vi "Pressure_Test_V2.vi"() -> ()   [LabVIEW 2015]
uses:
  <vilib>/Waveform/WDTOps.llb/WDT Append Waveforms DBL.vi
  <vilib>/Waveform/WDTOps.llb/WDT Waveform Duration DBL.vi
panel:
  in  "Stop Duration":dbl
  out "Current Duration":dbl format="%0.2f"
  out "Waveform Chart 1":dynamicdata(graph)
  in  "Enable":bool=TRUE
  in  "Filename":path=path "VehicleAccerometer/Front_Left_ACC.lvm"
  in  "Data Collection":bool
  in  "number of samples":i32=800
  in  "rate":dbl=2000.0
  # "256"
  # "512"
  # "Accelerometer Settings"
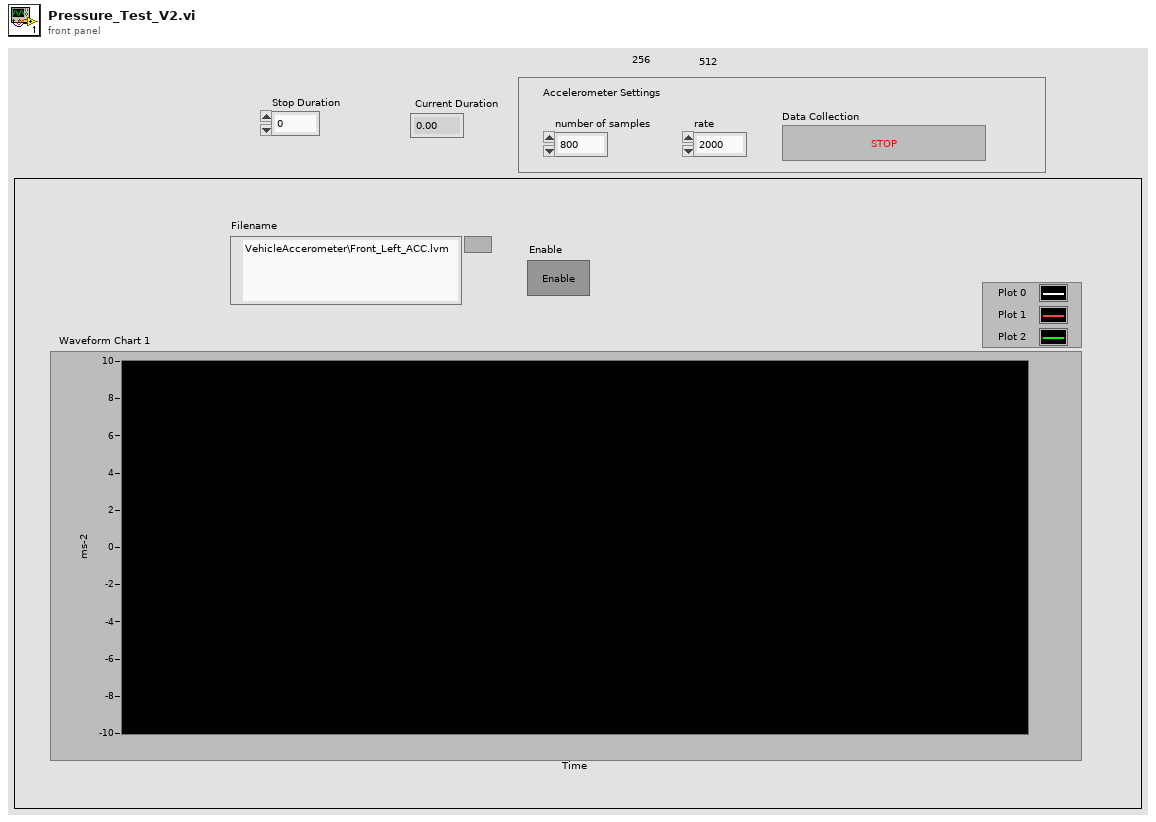
[diagram p1: front panel]
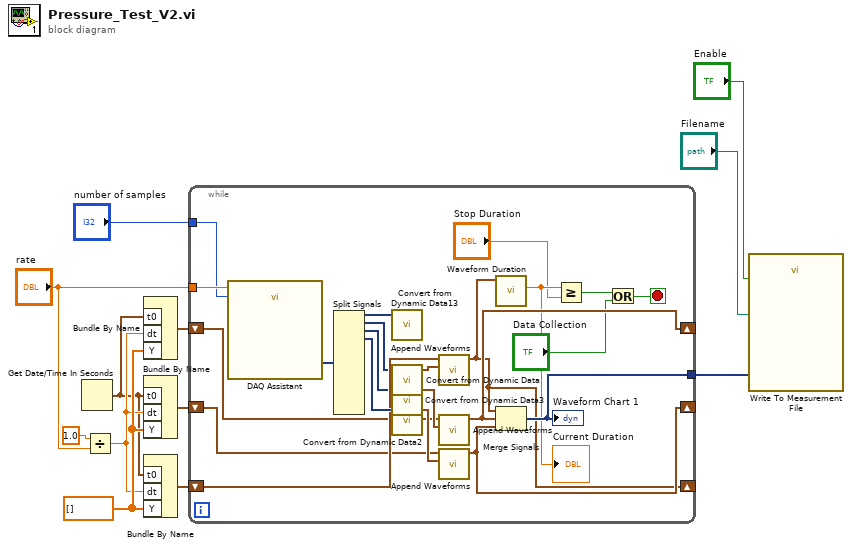
[diagram p0: block diagram]
diagram:
  w3 = dbl[] [] ("Y")
  n1 = Get Date/Time In Seconds() -> (seconds since 1Jan1904=w1:timestamp)
  n2 = Divide(x=1.0, y="rate") -> (x/y=w2:dbl)
  n3 = Bundle By Name("t0"=w1, "dt"=w2, "Y"=w3) -> (w12:waveform(dbl))  [unwired: 1 in]
  n4 = Bundle By Name("t0"=w1, "dt"=w2, "Y"=w3) -> (w9:waveform(dbl))  [unwired: 1 in]
  n5 = Bundle By Name("t0"=w1, "dt"=w2, "Y"=w3) -> (w8:waveform(dbl))  [unwired: 1 in]
  n6 = while {
    shift-right: [w23] -> _
    shift-left: w12 -> [w25]
    tunnel: "rate" -> [w31]
    shift-right: [w22] -> _
    shift-left: w9 -> [w24]
    shift-right: [w15] -> _
    shift-left: w8 -> [w28]
    tunnel: [w21] -> w5
    tunnel: "number of samples" -> [w14]
    stop <- w16 stop-if-true
    n7 = call "DAQ Assistant"("rate"=w31, "number of samples"=w14) -> ("data"=w30:dynamicdata)  [unwired: 15 in, 2 out]
    n8 = Split Signals(w30) -> (w13:dynamicdata, w26:dynamicdata, w27:dynamicdata, w34:dynamicdata)  [unwired: 13 in, 9 out]
    n9 = call "Convert from Dynamic Data13"("Dynamic Data Type"=w13) -> ()  [unwired: 3 in, 1 out]
    n10 = call "Convert from Dynamic Data"("Dynamic Data Type"=w26) -> ("Waveform"=w29:waveform(dbl))  [unwired: 3 in]
    n11 = call "Convert from Dynamic Data3"("Dynamic Data Type"=w27) -> ("Waveform"=w33:waveform(dbl))  [unwired: 3 in]
    n12 = call "Convert from Dynamic Data2"("Dynamic Data Type"=w34) -> ("Waveform"=w32:waveform(dbl))  [unwired: 3 in]
    n13 = call-poly <vilib>:"Append Waveforms.vi"("waveform B"=w29, "waveform A"=w28) -> ("waveform out"=w15:waveform(dbl))  [unwired: 8 in, 1 out]
    n14 = call-poly <vilib>:"Append Waveforms.vi"("waveform B"=w33, "waveform A"=w25) -> ("waveform out"=w23:waveform(dbl))  [unwired: 8 in, 1 out]
    n15 = call-poly <vilib>:"Append Waveforms.vi"("waveform B"=w32, "waveform A"=w24) -> ("waveform out"=w22:waveform(dbl))  [unwired: 8 in, 1 out]
    n16 = call-poly <vilib>:"Waveform Duration.vi"("waveform in"=w15) -> ("duration"=w20:dbl)  [unwired: 8 in, 2 out]
    "Current Duration" <- w20
    n17 = Merge Signals(w15, w23, w22) -> (w21:dynamicdata)
    "Waveform Chart 1" <- w21
    n18 = Greater Or Equal?(x=w20, y="Stop Duration") -> (x >= y?=w18:bool)
    n19 = Or(x=w18, y="Data Collection") -> (x .or. y?=w16:bool)
  }
  n20 = call "Write To Measurement File"("Signals"=w5, "Enable"="Enable", "Filename"="Filename") -> ()  [unwired: 14 in, 3 out]
